vi "Read and Save as TDMS (Single Channel).vi"(0 "VISA resource name":refnum<visa-resource-name>, 1 "Segment Index (0)":i32 format="%.0g", 2 "TDMS Path":path, 5 "Measurement Source (1: Channel 1)":i32(ring)=1 items=["Channel 1"=1, "Channel 2"=2, "Channel 3"=3, "Channel 4"=4, "Function 1"=5, "Function 2"=6, "Function 3"=7, "Function 4"=8, "Memory 1"=9, "Memory 2"=10, "Memory 3"=11, "Memory 4"=12], 7 "Number of Samples (1000)":i32=1000, 9 "Maximum Time (10000ms)":u32=10000, 11 "error in (no error)":errorcluster, 12 "Offset (0)":i32, 13 "Waveform Format (0: Int8)":u16(ring) items=["Int8", "Int16", "Double"]) -> (4 "VISA resource name out":refnum<visa-resource-name>, 6 "Waveform Information":T1, 10 "Written Samples":i32, 15 "error out":errorcluster)   [LabVIEW 2013, in "Agilent 90000 Series.lvlib"]
doc: "Returns scaled/unscaled data points of single channel from the instrument and save them into a TDMS file on the specified format."
uses:
  Agilent 90000 Series.lvlib
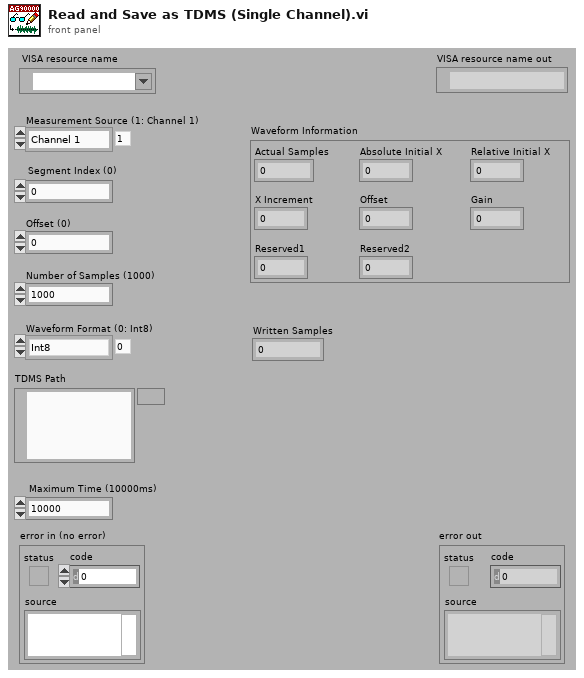
[diagram p1: front panel]
types:
  T1 = cluster{"Actual Samples":i32, "Absolute Initial X":dbl, "Relative Initial X":dbl, "X Increment":dbl, "Offset":dbl, "Gain":dbl, "Reserved1":dbl, "Reserved2":dbl}
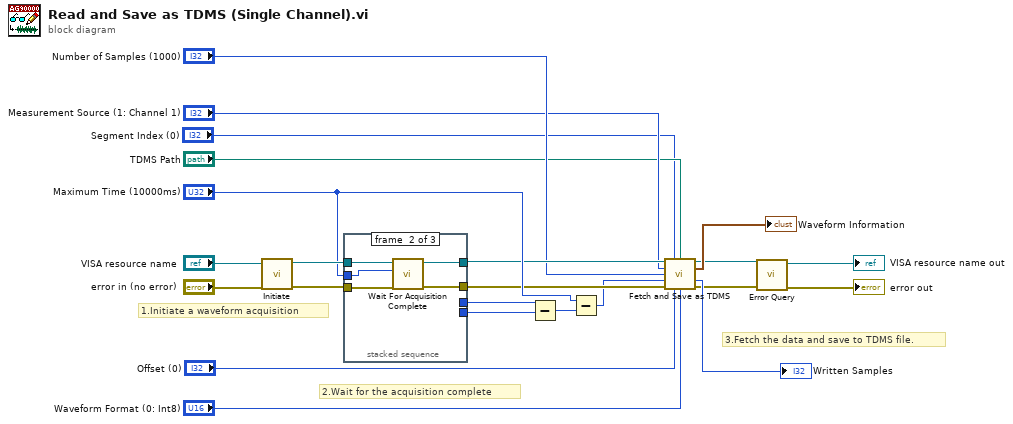
[diagram p0: block diagram]
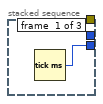
[diagram p2: hidden frame]
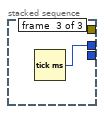
[diagram p3: hidden frame]
diagram:
  # "3.Fetch the data and save to TDMS file."
  # "2.Wait for the acquisition complete"
  # "1.Initiate a waveform acquisition"
  n1 = call "Initiate.vi"("error in (no error)"="error in (no error)", "VISA resource name"="VISA resource name") -> ("error out"=w20:errorcluster, "VISA resource name out"=w21:refnum<visa-resource-name>)  [unwired: 8 out]
  n2 = stacked-sequence {
    tunnel: [w24 _ _] -> w16
    tunnel: [_ _ w30] -> w17
    tunnel: w21 -> [_ w26 _]
    tunnel: [_ w29 _] -> w15
    tunnel: w20 -> [_ w27 _]
    tunnel: [_ w28 _] -> w14
    tunnel: "Maximum Time (10000ms)" -> [_ w25 _]
    frame #0 {
      n3 = Tick Count (ms)() -> (millisecond timer value=w24:u32)
    }
    frame #1 {
      n4 = call "Wait For Acquisition Complete.vi"("error in (no error)"=w27, "Maximum Time (10000ms)"=w25, "VISA resource name"=w26) -> ("error out"=w28:errorcluster, "VISA resource name out"=w29:refnum<visa-resource-name>)  [unwired: 7 out]
    }
    frame #2 {
      n5 = Tick Count (ms)() -> (millisecond timer value=w30:u32)
    }
  }
  n6 = Subtract(x=w17, y=w16) -> (x-y=w19:u32)
  n7 = Subtract(x="Maximum Time (10000ms)", y=w19) -> (x-y=w11:u32)
  n8 = call "Fetch and Save as TDMS.vi"("VISA resource name"=w15, "Segment Index (0)"="Segment Index (0)", "TDMS Path"="TDMS Path", "Measurement Source (1: Channel 1)"="Measurement Source (1: Channel 1)", "Number of Samples (1000)"="Number of Samples (1000)", "Maximum Time (10000ms)"=w11, "error in (no error)"=w14, "Offset (0)"="Offset (0)", "Waveform Format (0: Int8)"="Waveform Format (0: Int8)") -> ("VISA resource name out"=w4:refnum<visa-resource-name>, "Waveform Information"=→"Waveform Information":T1, "Written Samples"=→"Written Samples":i32, "error out"=w3:errorcluster)  [unwired: 3 out]
  n9 = call "Error Query.vi"("error in (no error)"=w3, "VISA resource name"=w4) -> ("error out"=→"error out":errorcluster, "VISA resource name out"=→"VISA resource name out":refnum<visa-resource-name>)  [unwired: 8 out]
